vi "_USB_CAN_BOARD_INFO_.vi"(11 "VCI_BOARD_INFO":T1) -> ()   [LabVIEW 2011]
panel:
  in  "ok":bool
  out "str_hw_Type":string caption="硬件类型："
  out "str_Serial_Num":string caption="板卡序列号："
  out "can_Num":u8 caption="can通道数："
  out "irq_Num":u16 caption="板载中断：" format="0x%x"
  out "in_Ver":string caption="动态库版本："
  out "dr_Ver":string caption="驱动版本："
  out "fw_Ver":string caption="固件版本："
  out "hw_Ver":string caption="硬件版本："
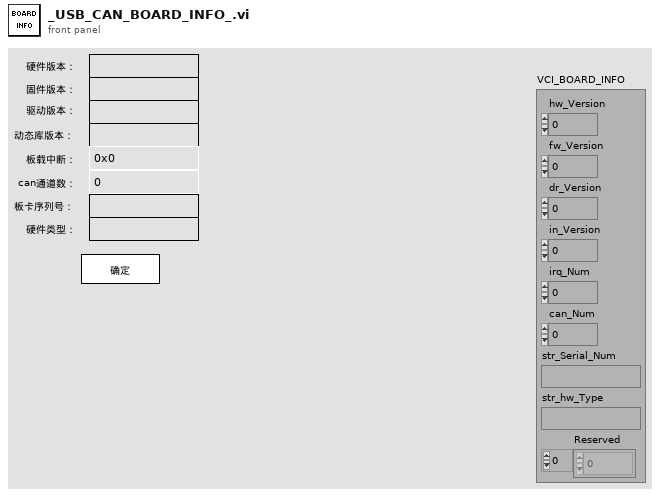
[diagram p1: front panel]
types:
  T1 = cluster{"hw_Version":u16, "fw_Version":u16, "dr_Version":u16, "in_Version":u16, "irq_Num":u16, "can_Num":u8, "str_Serial_Num":string, "str_hw_Type":string, "Reserved":u8[]}
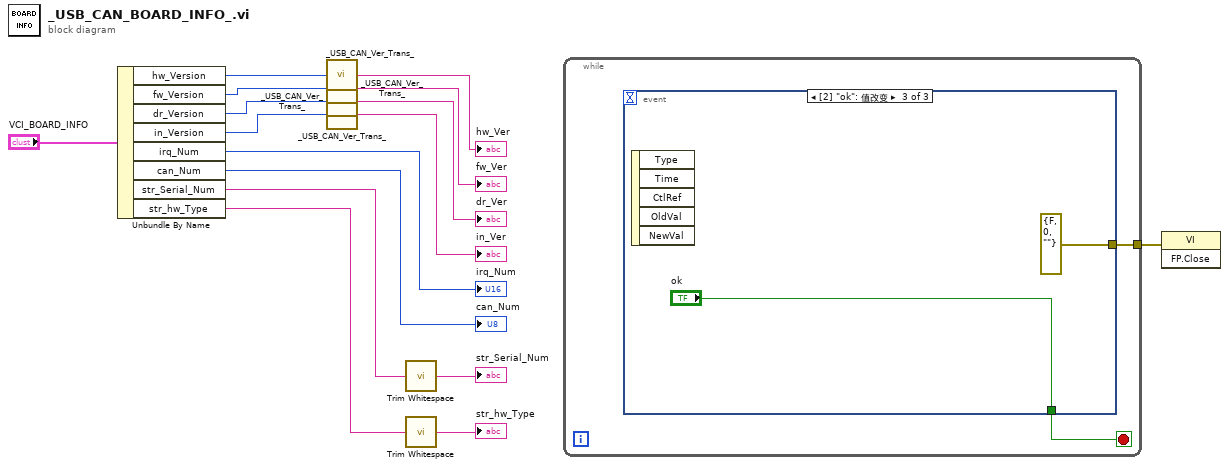
[diagram p0: block diagram]
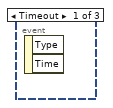
[diagram p2: hidden frame]
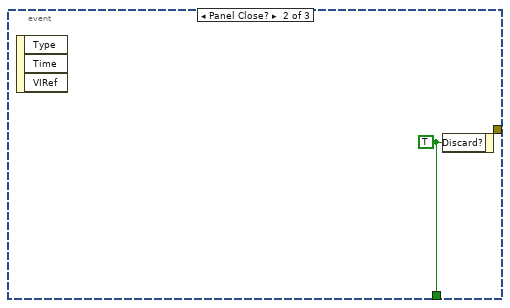
[diagram p3: hidden frame]
diagram:
  n1 = Unbundle By Name("VCI_BOARD_INFO") -> ("hw_Version"=w10:u16, "fw_Version"=w9:u16, "dr_Version"=w8:u16, "in_Version"=w7:u16, "irq_Num"=→"irq_Num":u16, "can_Num"=→"can_Num":u8, "str_Serial_Num"=w3:string, "str_hw_Type"=w1:string)
  n2 = call "_USB_CAN_Ver_Trans_.vi"("u16Ver"=w10) -> ("strVer"=→"hw_Ver":string)
  n3 = call "_USB_CAN_Ver_Trans_.vi"("u16Ver"=w9) -> ("strVer"=→"fw_Ver":string)
  n4 = call "_USB_CAN_Ver_Trans_.vi"("u16Ver"=w8) -> ("strVer"=→"dr_Ver":string)
  n5 = call "_USB_CAN_Ver_Trans_.vi"("u16Ver"=w7) -> ("strVer"=→"in_Ver":string)
  n6 = call <vilib>:"Trim Whitespace.vi"("string"=w3) -> ("trimmed string"=→"str_Serial_Num":string)  [unwired: 1 in]
  n7 = call <vilib>:"Trim Whitespace.vi"("string"=w1) -> ("trimmed string"=→"str_hw_Type":string)  [unwired: 1 in]
  n8 = while {
    tunnel: [w17] -> w16
    stop <- w18 stop-if-true
    n9 = event shown="[2] \"ok\": 值改变" {
      selector: _ -> [_ _ _]
      dyn-events: _ -> [_ _ _]
      timeout: _ -> [_ _ _]
      tunnel: [_ w19 "ok"] -> w18
      tunnel: [_ _ errorcluster {"status"=FALSE, "code"=0, "source"=""} ("错误输入（无错误）")] -> w17
      event Timeout {
        n10 = event-data() -> ()  [unwired: 1 in, 2 out]
      }
      event Panel Close? {
        w19 = TRUE ("放弃？")
        n11 = event-data() -> ()  [unwired: 1 in, 3 out]
        n12 = event-data("Discard?"=w19) -> ()  [unwired: 1 in, 1 out]
      }
      event "ok": Value Change {
        n13 = event-data() -> ()  [unwired: 1 in, 5 out]
      }
    }
  }
  n14 = invoke class="VI" method="FP.Close"(error in=w16) -> ()  [unwired: 2 in, 3 out]
